vi "DAQNavi Read (Analog 2D DBL NChan NSamp).vi"(8 "error in (no error)":errorcluster, 9 "number of samples per channel to read":u32=1000, 10 "timeout":dbl=10.0 format="%0.2f", 11 "task in":i32) -> (0 "error out":errorcluster, 1 "markBuf":cluster{"Data Index":i64, "Src Id":i64}[](array[cluster]), 2 "data":dbl[][](array[numeric]), 3 "task out":i32)   [LabVIEW 2020]
uses:
  DAQNavi_LV.dll
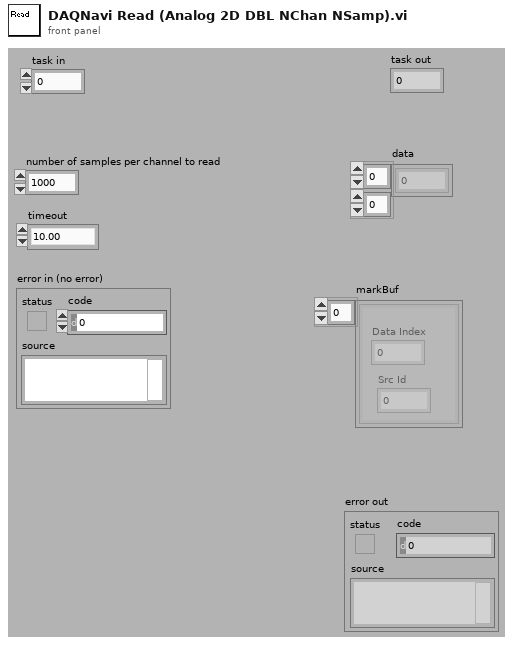
[diagram p1: front panel]
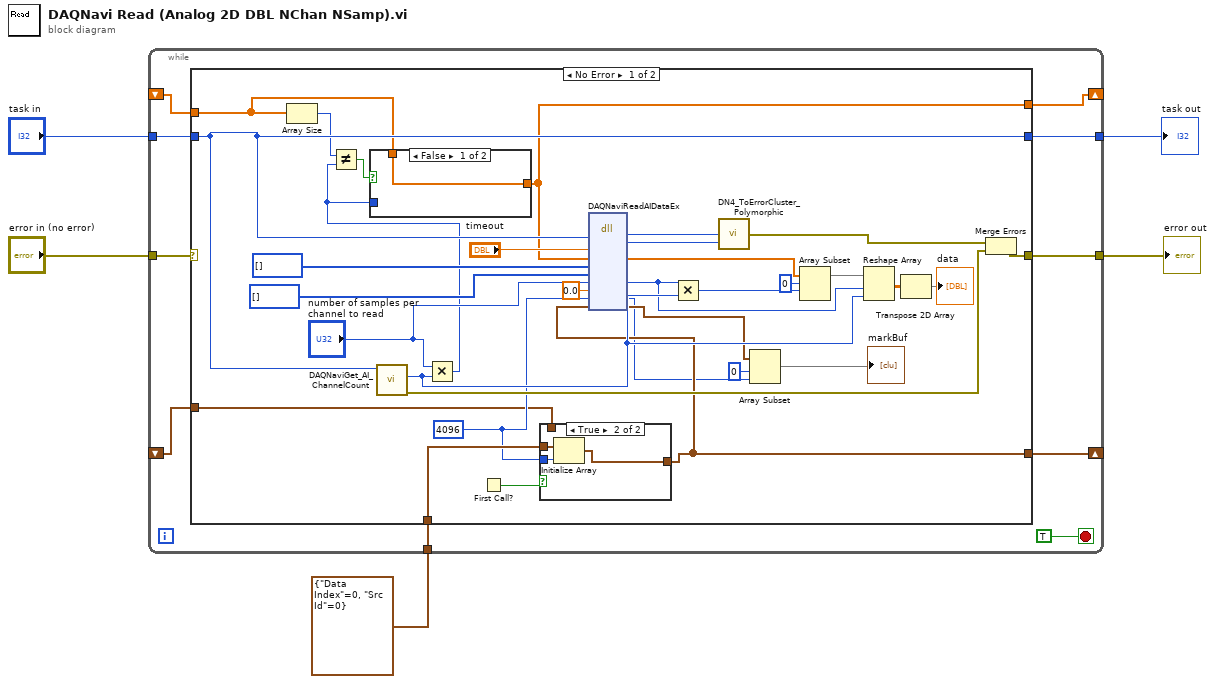
[diagram p0: block diagram]
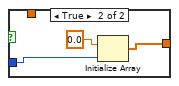
[diagram p3: hidden frame]
diagram:
  n1 = while {
    tunnel: "task in" -> [w15]
    tunnel: "error in (no error)" -> [w14]
    tunnel: [w13] -> w3
    tunnel: [w12] -> w2
    shift-right: [w10] -> _
    shift-left: _ -> [w9]
    tunnel: cluster{"Data Index":i64, "Src Id":i64} {"Data Index"=0, "Src Id"=0} -> [w8]
    shift-right: [w7] -> _
    shift-left: _ -> [w6]
    stop <- TRUE stop-if-true
    n2 = case shown="No Error" w14 {
      selector: w14 -> [_ w59]
      tunnel: w15 -> [w45 w60]
      tunnel: [w45 w60] -> w13
      tunnel: [w44 w59] -> w12
      tunnel: [w30 w58] -> w10
      tunnel: w9 -> [w26 w58]
      tunnel: w8 -> [w25 _]
      tunnel: [w21 w57] -> w7
      tunnel: w6 -> [w22 w57]
      frame No Error {
        w24 = 4096
        n3 = Array Size(array=w26) -> (size(s)=w28:i32)
        n4 = call "DAQNaviGet_AI_ChannelCount.vi"("task in"=w45) -> ("error out"=w42:errorcluster, "channel count"=w37:i32)  [unwired: 1 in, 8 out]
        n5 = Multiply(x="number of samples per channel to read", y=w37) -> (x*y=w27:u32)
        n6 = Not Equal?(x=w28, y=w27) -> (x != y?=w29:bool)
        n7 = case shown="False" w29 {
          tunnel: [w53 w55] -> w30
          tunnel: w27 -> [_ w54]
          tunnel: w26 -> [w53 _]
          frame False {
          }
          frame True {
            n8 = Initialize Array(0.0 ("element"), w54) -> (w55:dbl[])
          }
        }
        n9 = First Call?() -> (First Call?: T/F=w23:bool)
        n10 = case shown="True" w23 {
          tunnel: w25 -> [_ w52]
          tunnel: w24 -> [_ w51]
          tunnel: [w49 w50] -> w21
          tunnel: w22 -> [w49 _]
          frame False {
          }
          frame True {
            n11 = Initialize Array(w52, w51) -> (w50:cluster{"Data Index":i64, "Src Id":i64}[])
          }
        }
        n12 = dll-call lib="DAQNavi_LV.dll" fn="DAQNaviReadAIDataEx"("taskID"=w45, "timeout"="timeout", "scaledData"=w30, "rawData16"=u16[] [] ("rawData32"), "rawData32"=u32[] [] ("scaledData"), "samples"="number of samples per channel to read", "startTime"=0.0, "markCount"=w24, "markBuf"=w21) -> ("return type"=w47:i32, "taskID"=w31:i32, "scaledData"=w33:dbl[], "samples"=w36:u32, "markCount"=w19:i32, "markBuf"=w20:cluster{"Data Index":i64, "Src Id":i64}[])  [unwired: 4 in, 5 out]
        n13 = Multiply(x=w36, y=w37) -> (x*y=w38:u32)
        n14 = call "DN4_ToErrorCluster_Polymorphic.vi"("task id"=w31, "error code"=w47) -> ("error out"=w43:errorcluster)  [unwired: 3 out]
        n15 = Array Subset(array=w20, index=0, length=w19) -> (→"markBuf":cluster{"Data Index":i64, "Src Id":i64}[])
        n16 = Array Subset(array=w33, index=0, length=w38) -> (w41:dbl[])
        n17 = Reshape Array(w41, w36, w37) -> (w40:dbl[][])
        n18 = Transpose 2D Array(2D array=w40) -> (transposed array=→"data":dbl[][])
        n19 = Merge Errors(w43, w42) -> (w44:errorcluster)
      }
      frame Error {
      }
    }
  }
  "task out" <- w3
  "error out" <- w2
